vi "ex_3a.vi"() -> ()   [LabVIEW 2020]
uses:
  <vilib>/numeric/Random Number (Range) U64.vi
  <vilib>/numeric/sub_Random U32.vi
panel:
  out "Array K":u64[](array[numeric])
  out "Array M":u64[](array[numeric])
  out "Result":u64[](array[numeric])
  in  "K":i32
  in  "M":i32
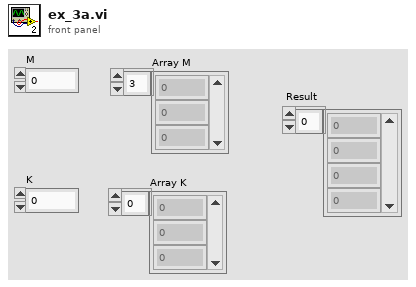
[diagram p1: front panel]
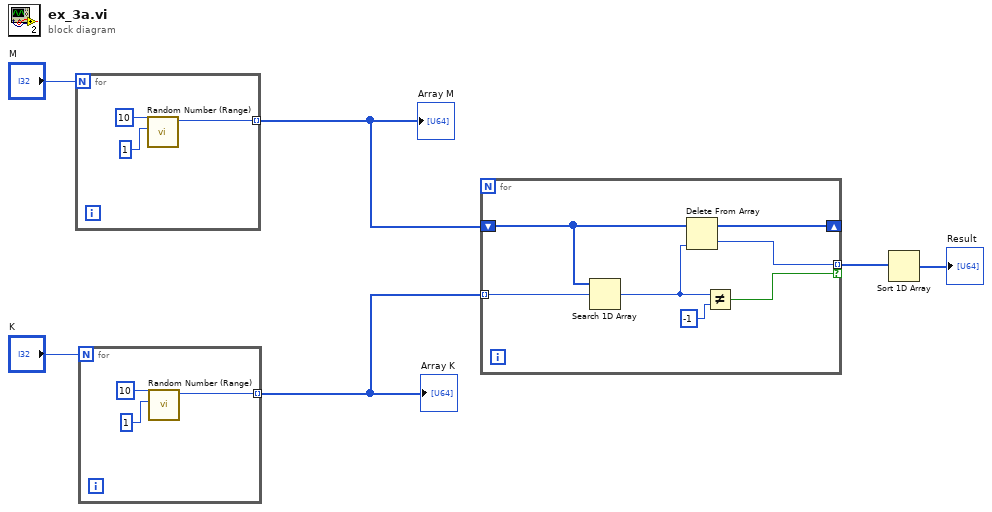
[diagram p0: block diagram]
diagram:
  n1 = for {
    N: "M" -> [_]
    tunnel: [w7] -> w3 mode=indexing
    n2 = call-poly <vilib>:"Random Number (Range).vi"("lower bound (0)"=u64 1, "upper bound (100)"=u64 10) -> ("number"=w7:u64)  [unwired: 9 in]
  }
  "Array M" <- w3
  n3 = for {
    N: "K" -> [_]
    tunnel: [w10] -> w4 mode=indexing
    n4 = call-poly <vilib>:"Random Number (Range).vi"("lower bound (0)"=u64 1, "upper bound (100)"=u64 10) -> ("number"=w10:u64)  [unwired: 9 in]
  }
  "Array K" <- w4
  n5 = for {
    tunnel: w4 -> [w19] mode=indexing
    shift-right: [w17] -> _
    shift-left: w3 -> [w18]
    tunnel: [w14] -> w2 mode=indexing if=w13
    n6 = Search 1D Array(1D array=w18, element=w19) -> (index of element=w16:i32)  [unwired: 1 in]
    n7 = Delete From Array(array=w18, index=w16) -> (deleted portion=w14:u64, array with subset deleted=w17:u64[])  [unwired: 1 in]
    n8 = Not Equal?(x=w16, y=-1) -> (x != y?=w13:bool)
  }
  n9 = Sort 1D Array(array=w2) -> (sorted array=→"Result":u64[])
